vi "ztscopeM Horizontal Query.vi"(8 "error in":errorcluster, 11 "Instrument Handle In":i32) -> (0 "error out":errorcluster, 1 "Sample Time":dbl, 2 "Sample Points":u32, 3 "Instrument Handle Out":i32, 4 "Offset Time":dbl)   [LabVIEW 2013]
doc: "Query the horizontal and timebase settings."
uses:
  ztscopeM.dll
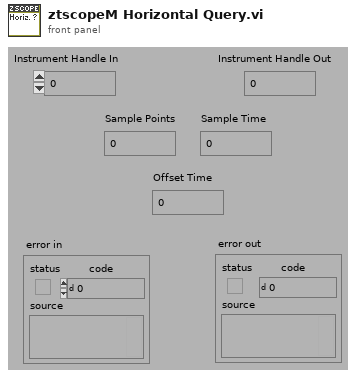
[diagram p1: front panel]
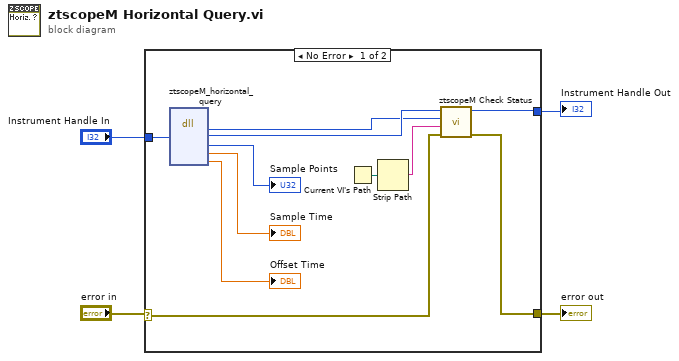
[diagram p0: block diagram]
diagram:
  n1 = case shown="No Error" "error in" {
    selector: "error in" -> [w7 w17]
    tunnel: [w6 w17] -> w1
    tunnel: "Instrument Handle In" -> [w15 w16]
    tunnel: [w5 w16] -> w3
    frame No Error {
      n2 = dll-call lib="C:/Program Files/National Instruments/instr.lib/ztscopem/ztscopeM.dll" fn="ztscopeM_horizontal_query"("instrumentHandle"=w15) -> (w8:i32, "instrumentHandle"=w9:i32, "samplePoints"=→"Sample Points":u32, "sampleTime"=→"Sample Time":dbl, "offsetTime"=→"Offset Time":dbl)  [unwired: 6 in, 2 out]
      n3 = Current VI's Path() -> (path=w11:path)
      n4 = Strip Path(path=w11) -> (name=w10:string)  [unwired: 1 out]
      n5 = call "ztscopeM Check Status.vi"("error in"=w7, "name of VI"=w10, "status"=w8, "instrument handle in"=w9) -> ("error out"=w6:errorcluster, "instrument handle out"=w5:i32)  [unwired: 2 in]
    }
    frame Error {
    }
  }
  "Instrument Handle Out" <- w3
  "error out" <- w1
